vi "Set Panel Controls and VI Ref.vi"(8 "error in (no error)":errorcluster, 10 "Controls and VI Refnum":T1, 11 "Panel View.lvclass":refnum<class "Panel View.lvclass">) -> (0 "error out":errorcluster, 3 "Panel View.lvclass Out":refnum<class "Panel View.lvclass">)   [LabVIEW 2015, in "Panel View.lvclass"]
uses:
  Panel View.lvclass
  Panel Manager/Type Definition/Controls and VI Refnums.ctl
  Panel View.lvclass/Panel View.ctl
  Panel Manager/Panel Manager Controller.lvclass
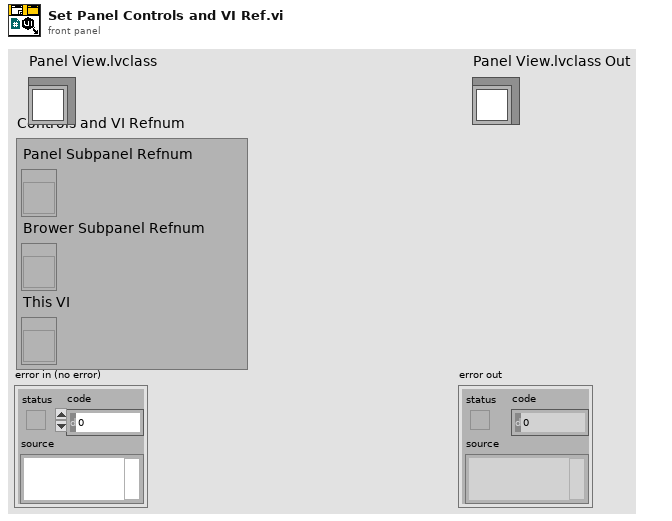
[diagram p1: front panel]
types:
  T1 = typedef "Panel Manager Controller.lvclass/Controls and VI Refnums.ctl" = cluster{"Panel Subpanel Refnum":refnum<vi>, "Brower Subpanel Refnum":refnum<vi>, "This VI":refnum<vi>}
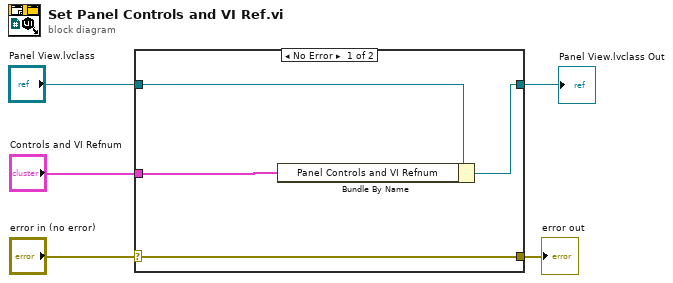
[diagram p0: block diagram]
diagram:
  n1 = case shown="No Error" "error in (no error)" {
    selector: "error in (no error)" -> [w9 w10]
    tunnel: [w9 w10] -> w4
    tunnel: [w7 w11] -> w1
    tunnel: "Panel View.lvclass" -> [w8 w11]
    tunnel: "Controls and VI Refnum" -> [w6 _]
    frame No Error {
      n2 = Bundle By Name(cluster=w8, "Panel Controls and VI Refnum"=w6) -> (w7:refnum<class "Panel View.lvclass">)
    }
    frame Error {
    }
  }
  "error out" <- w4
  "Panel View.lvclass Out" <- w1
